vi "getType.vi"(8 "error in (no error)":errorcluster, 11 "Generic In":refnum<class "Generic.lvclass">) -> (0 "error out":errorcluster, 2 "type":string, 3 "Generic Out":refnum<class "Generic.lvclass">)   [LabVIEW 2023, in "TLC_Scripto.lvlib" / "Generic.lvclass"]
uses:
  Generic.lvclass
  <vilib>/regexp/Match Regular Expression.xnode
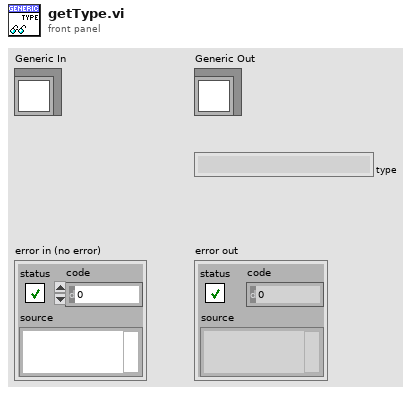
[diagram p1: front panel]
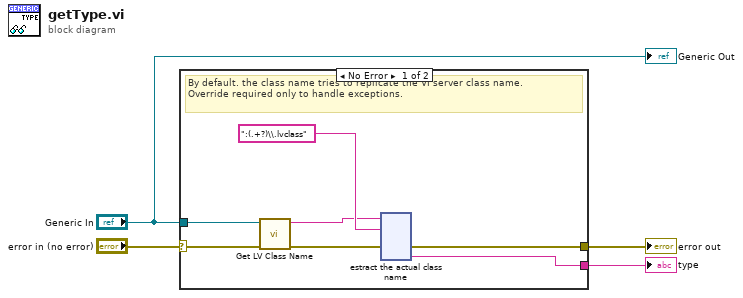
[diagram p0: block diagram]
diagram:
  n1 = case shown="No Error" "error in (no error)" {
    selector: "error in (no error)" -> [w11 w131]
    tunnel: "Generic In" -> [w10 _]
    tunnel: [w7 _] -> w3
    tunnel: [w5 w131] -> w1
    frame No Error {
      # "By default. the class name tries to replicate the VI server class name.\nOverride required only to handle exceptions."
      n2 = call <vilib>:"Get LV Class Name.vi"("error in (no error)"=w11, "object"=w10) -> ("error out"=w6:errorcluster, "class name"=w8:string)  [unwired: 8 in]
      n3 = xnode "estract the actual class name"("input string"=w8, "regular expression"=":(.+?)\\.lvclass", "error in"=w6) -> ("error out"=w5:errorcluster, "submatch 1"=w7:string)  [unwired: 3 in, 4 out]
    }
    frame Error {
    }
  }
  "error out" <- w1
  "type" <- w3
  "Generic Out" <- "Generic In"
